vi "ZCAN_ClearBuffer.vi"(8 "error in (no error)":errorcluster, 11 "can_index_handle":u32) -> (0 "error out":errorcluster, 3 "ClearBuffer_success?":bool)   [LabVIEW 2020, in "zlgcan.lvlib"]
uses:
  zlgcan.lvlib
  bin/zlgcan_wrap.dll
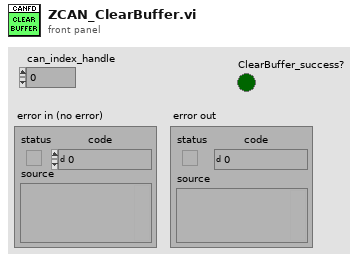
[diagram p1: front panel]
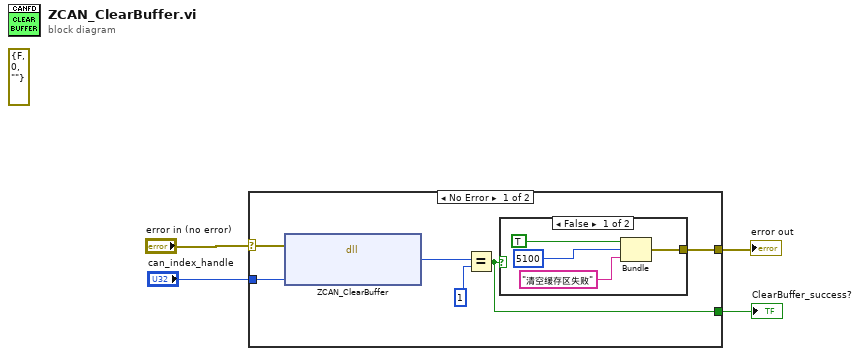
[diagram p0: block diagram]
diagram:
  (unwired) errorcluster {"status"=FALSE, "code"=0, "source"=""} ("error out")
  n1 = case shown="No Error" "error in (no error)" {
    selector: "error in (no error)" -> [w5 w15]
    tunnel: [w8 w15] -> w2
    tunnel: "can_index_handle" -> [w10 _]
    tunnel: [w6 _] -> w3
    frame No Error {
      n2 = dll-call lib="E:/Jabil tools/JabilTestLib/ZLG_CANFD/bin/zlgcan_wrap.dll" fn="ZCAN_ClearBuffer" ("ZCAN_StartCAN")(error in=w5, "can_handle"=w10) -> ("return"=w7:u32)  [unwired: 3 in, 2 out]
      n3 = Equal?(x=w7, y=1) -> (x = y?=w6:bool)
      n4 = case shown="False" w6 {
        tunnel: [w11 _] -> w8
        frame False {
          n5 = Bundle("status"=TRUE, "code"=5100, "消息"="清空缓存区失败") -> (w11:cluster{"status":bool, "code":i32, "消息":string})  [unwired: 1 in]
        }
        frame True {
        }
      }
    }
    frame Error {
    }
  }
  "ClearBuffer_success?" <- w3
  "error out" <- w2
